vi "AD7609 sleepmode.vi"(1 "Sleep state":u8(ring) items=["Awake", "Standby", "Shutdown"]) -> (0 "Sleep error out":errorcluster)   [LabVIEW 2014]
uses:
  <vilib>/Instr/_visa.llb/VISA Open Access Mode.ctl
  <vilib>/Instr/_visa.llb/VISA Configure Serial Port (Instr).vi
  AD7609 global.vi
panel:
  out "Sleep string output":string
  # "PN 25/11/2014"
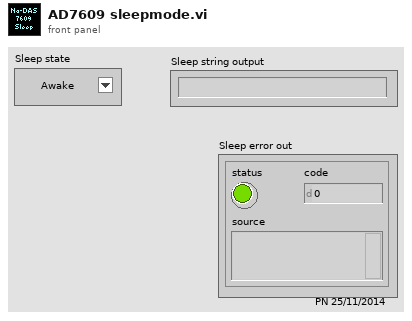
[diagram p1: front panel]
types:
  T1 = typedef "VISA Open Access Mode.ctl" = u32
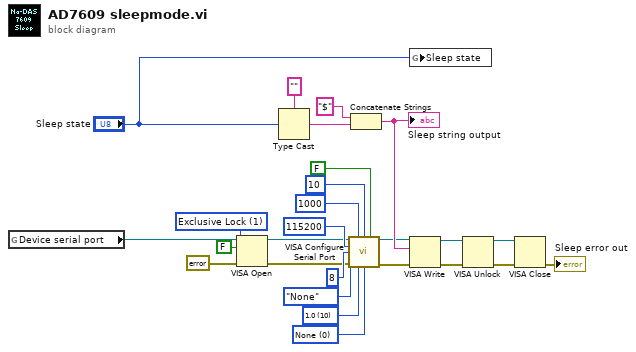
[diagram p0: block diagram]
diagram:
  w14 = T1 1 items=["VISA Defaults"=0, "Exclusive Lock"=1, "Load Configured Settings"=4] ("Access Mode")
  w15 = u16 0 items=["None", "XON/XOFF", "RTS/CTS", "XON/XOFF & RTS/CTS", "DTR/DSR", "XON/XOFF & DTR/DSR"] ("flow control (0:none)")
  w16 = u16 10 items=["1.0"=10, "1.5"=15, "2.0"=20] ("stop bits (10: 1 bit)")
  n1 = global read "AD7609 global.vi" "Device serial port"() -> (w2:refnum<visa-resource-name>)
  n2 = VISA Open(duplicate session (F)=FALSE, access mode=w14, error in (no error)=errorcluster {"status"=FALSE, "code"=0, "source"=""}, VISA resource name=w2) -> (VISA resource name=w5:refnum<visa-resource-name>, error out=w7:errorcluster)  [unwired: 1 in]
  n3 = Type Cast(type="", x="Sleep state") -> (*(type *) &x=w25:string)
  n4 = call-poly "VISA Configure Serial Port"("VISA resource name"=w5, "timeout (10sec)"=u32 1000, "termination char\n(0xA = '\\n' = LF)"=u8 10 ("termination char\n(0xA = '\\n' = LF)"), "Enable Termination\nChar (T)"=FALSE ("Enable Termination\nChar (T)"), "baud rate (9600)"=u32 115200, "data bits (8)"=u16 8, "parity (0:none)"=enum16{"None", "Odd", "Even", "Mark", "Space"}."None", "error in (no error)"=w7, "stop bits (10: 1 bit)"=w16, "flow control (0:none)"=w15) -> ("VISA resource name out"=w4:refnum<visa-resource-name>, "error out"=w6:errorcluster)  [unwired: 4 in]
  n5 = Concatenate Strings("$", w25) -> (w23:string)
  "Sleep string output" <- w23
  n6 = global write "AD7609 global.vi" "Sleep state"("Sleep state") -> ()
  n7 = VISA Write(VISA resource name=w4, write buffer=w23, error in (no error)=w6) -> (VISA resource name out=w9:refnum<visa-resource-name>, error out=w8:errorcluster)  [unwired: 1 out]
  n8 = VISA Unlock(8:w8, 11:w9) -> (0:w11:errorcluster, 3:w12:refnum<visa-resource-name>)
  n9 = VISA Close(VISA resource name=w12, error in (no error)=w11) -> (error out=→"Sleep error out":errorcluster)
